vi "overlay_particle_number(subVI).vi"(8 "error in (no error)":errorcluster, 10 "Particle Reports (Pixels)":T2(array[cluster]), 11 "Image":T1) -> (0 "error out":errorcluster, 3 "number of particle":i32)   [LabVIEW 2020]
uses:
  <vilib>/vision/Image Controls.llb/IMAQ Image.ctl
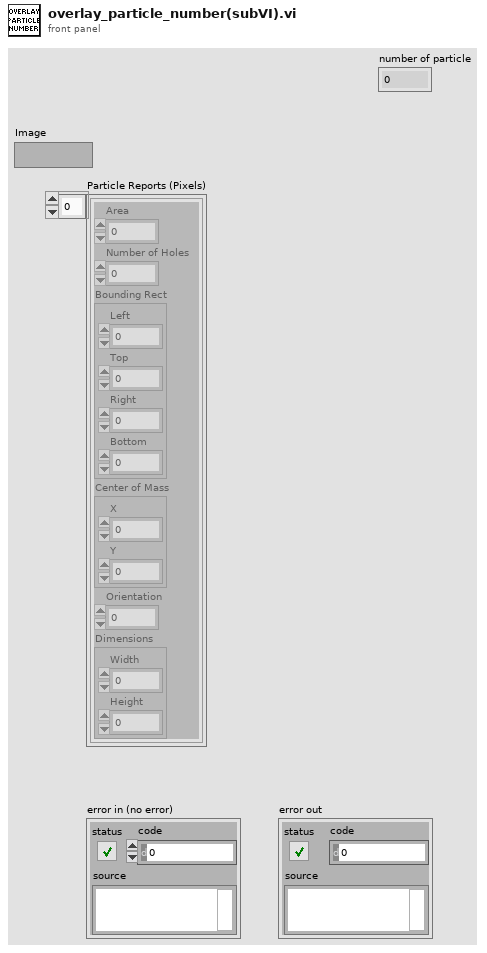
[diagram p1: front panel]
types:
  T1 = typedef "IMAQ Image.ctl" = refnum<image>
  T2 = cluster{"Area":dbl, "Number of Holes":dbl, "Bounding Rect":cluster{"Left":dbl, "Top":dbl, "Right":dbl, "Bottom":dbl}, "Center of Mass":cluster{"X":dbl, "Y":dbl}, "Orientation":dbl, "Dimensions":cluster{"Width":dbl, "Height":dbl}}[]
  T3 = cluster{"Desired Font (Application)":enum16{"User-specified Font", "Application Font", "System Font", "Dialog Font"}, "[User-specified Font]":cluster{"Font Name":string, "Size":i16, "Strikeout?":bool, "Italic?":bool, "Underline?":bool, "Outline?":bool, "Shadow?":bool, "Bold?":bool, "Rotation Angle":dbl}, "Horizontal Alignment":i16, "Vertical Alignment":i16}
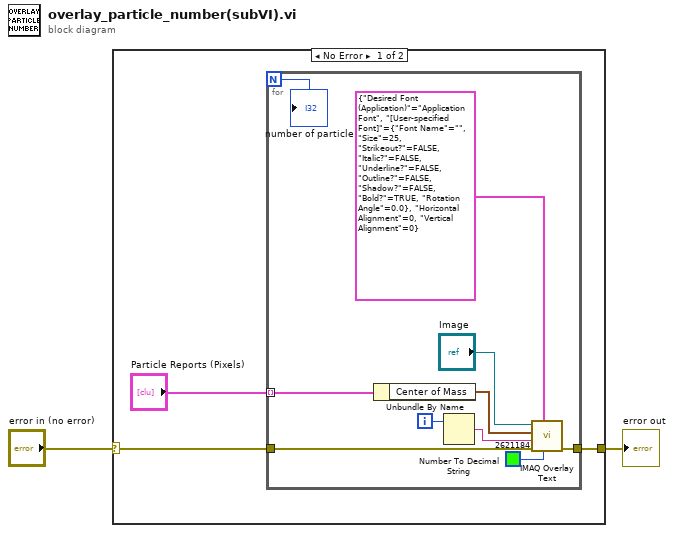
[diagram p0: block diagram]
diagram:
  n1 = case shown="No Error" "error in (no error)" {
    selector: "error in (no error)" -> [w3 w16]
    tunnel: [w5 w16] -> w2
    frame No Error {
      n2 = for {
        N -> [w6]
        tunnel: [w10] -> w5
        tunnel: "Particle Reports (Pixels)" -> [w8] mode=indexing
        tunnel: w3 -> [w7]
        i -> [w14]
        n3 = Unbundle By Name(w8) -> ("Center of Mass"=w15:cluster{"X":dbl, "Y":dbl})
        n4 = Number To Decimal String(number=w14) -> (decimal integer string=w13:string)  [unwired: 1 in]
        n5 = call "IMAQ Overlay Text"("Text Color (black)"=u32 2621184, "Font, Size & Style"=T3 {"Desired Font (Application)"=enum."Application Font", "[User-specified Font]"={"Font Name"="", "Size"=25, "Strikeout?"=FALSE, "Italic?"=FALSE, "Underline?"=FALSE, "Outline?"=FALSE, "Shadow?"=FALSE, "Bold?"=TRUE, "Rotation Angle"=0.0}, "Horizontal Alignment"=0, "Vertical Alignment"=0}, "error in (no error)"=w7, "String"=w13, "Origin"=w15, "Image"="Image") -> ("error out"=w10:errorcluster)  [unwired: 4 in, 1 out]
        "number of particle" <- w6
      }
    }
    frame Error {
    }
  }
  "error out" <- w2
